vi "OM3_OdorControl.vi"(1 "Odor#":i32) -> ()   [LabVIEW 2015]
uses:
  <vilib>/Instr/_visa.llb/VISA Configure Serial Port (Instr).vi
  <vilib>/Utility/file.llb/Read Delimited Spreadsheet (I64).vi
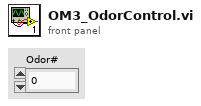
[diagram p1: front panel]
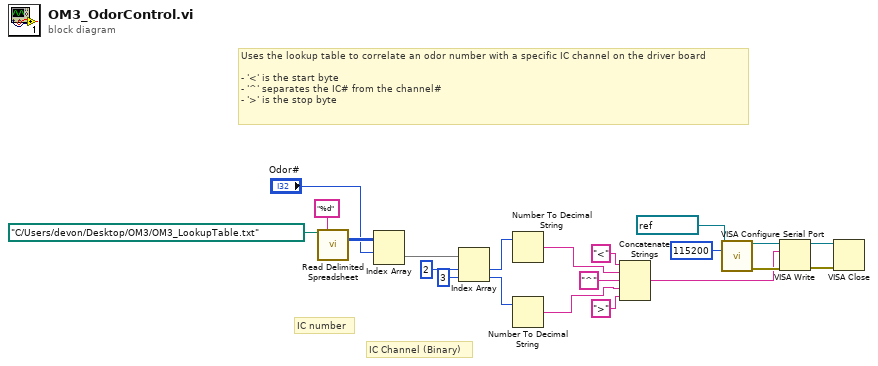
[diagram p0: block diagram]
diagram:
  # "IC Channel (Binary)"
  # "IC number"
  # "Uses the lookup table to correlate an odor number with a specific IC channel on the driver board\n\n- '<' is the start byte\n- '^' separates the IC# from the channel#\n- '>' is the stop byte"
  n1 = call-poly <vilib>:"Read Delimited Spreadsheet.vi"("file path (dialog if empty)"=path "C:/Users/devon/Desktop/OM3/OM3_LookupTable.txt", "format (%d)"="%d" ("format (%.3f)")) -> ("all rows"=w9:i64[][])  [unwired: 8 in, 5 out]
  n2 = Index Array(array=w9, index (row)="Odor#") -> (element=w7:i64[])  [unwired: 1 in]
  n3 = Index Array(array=w7, index #1=2 ("index"), index #2=3 ("index")) -> (element #1=w5:i64, element #2=w3:i64)
  n4 = Number To Decimal String(number=w5) -> (decimal integer string=w2:string)  [unwired: 1 in]
  n5 = Number To Decimal String(number=w3) -> (decimal integer string=w1:string)  [unwired: 1 in]
  n6 = Concatenate Strings("<" ("string"), w2, "^" ("string"), w1, ">" ("string")) -> (w12:string)
  n7 = call-poly "VISA Configure Serial Port"("VISA resource name"=refnum<visa-resource-name> "COM5", "baud rate (9600)"=u32 115200) -> ("VISA resource name out"=w19:refnum<visa-resource-name>, "error out"=w18:errorcluster)  [unwired: 12 in]
  n8 = VISA Write(VISA resource name=w19, write buffer=w12, error in (no error)=w18) -> (VISA resource name out=w16:refnum<visa-resource-name>, error out=w15:errorcluster)  [unwired: 1 out]
  n9 = VISA Close(VISA resource name=w16, error in (no error)=w15) -> ()  [unwired: 1 out]
